vi "GetCurrentThread (Standard).vi"(8 "error in (no error)":errorcluster, 11 "Impersonate in":refnum<class "LogonUser.lvclass">) -> (0 "error out":errorcluster, 1 "thread id":i64, 3 "Impersonate out":refnum<class "LogonUser.lvclass">)   [LabVIEW 2018, in "LogonUser.lvclass"]
doc: "©2019\nWiebe Walstra\nwww.carya.nl"
uses:
  LogonUser.lvclass
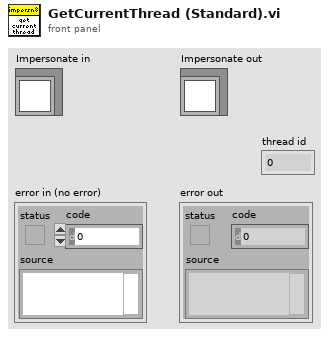
[diagram p1: front panel]
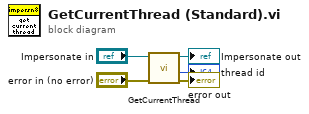
[diagram p0: block diagram]
diagram:
  n1 = call-dynamic "GetCurrentThread.vi"("error in (no error)"="error in (no error)", "Impersonate in"="Impersonate in") -> ("error out"=→"error out":errorcluster, "thread id"=→"thread id":i64, "Impersonate out"=→"Impersonate out":refnum<class "LogonUser.lvclass">)  [unwired: 7 in]
